vi "HW Run_20201229.vi"(8 "error in (no error)":errorcluster, 11 "ClusterOut in":T1) -> (0 "error out":errorcluster, 3 "ClusterOut out":T1)   [LabVIEW 2018]
uses:
  Controls/HWCluster.ctl
  Controls/Clusts/FPGA_Config_Clust.ctl
  Controls/Enums/TargetNumber.ctl
  Controls/Clusts/AcqData.ctl
  Controls/Clusts/SaturationMonitor.ctl
  Controls/Clusts/FromFPGA_Clust.ctl
  Queue/DataQueueElements.ctl
  Controls/Clusts/TimeDomainData.ctl
  Controls/Enums/LogLoopEnum.ctl
panel:
  out "Target1 2":i32
  out "Elements Remaining 3":u32
  out "Elements Remaining":u32
  out "Target 3":i32
  out "Target1":i32
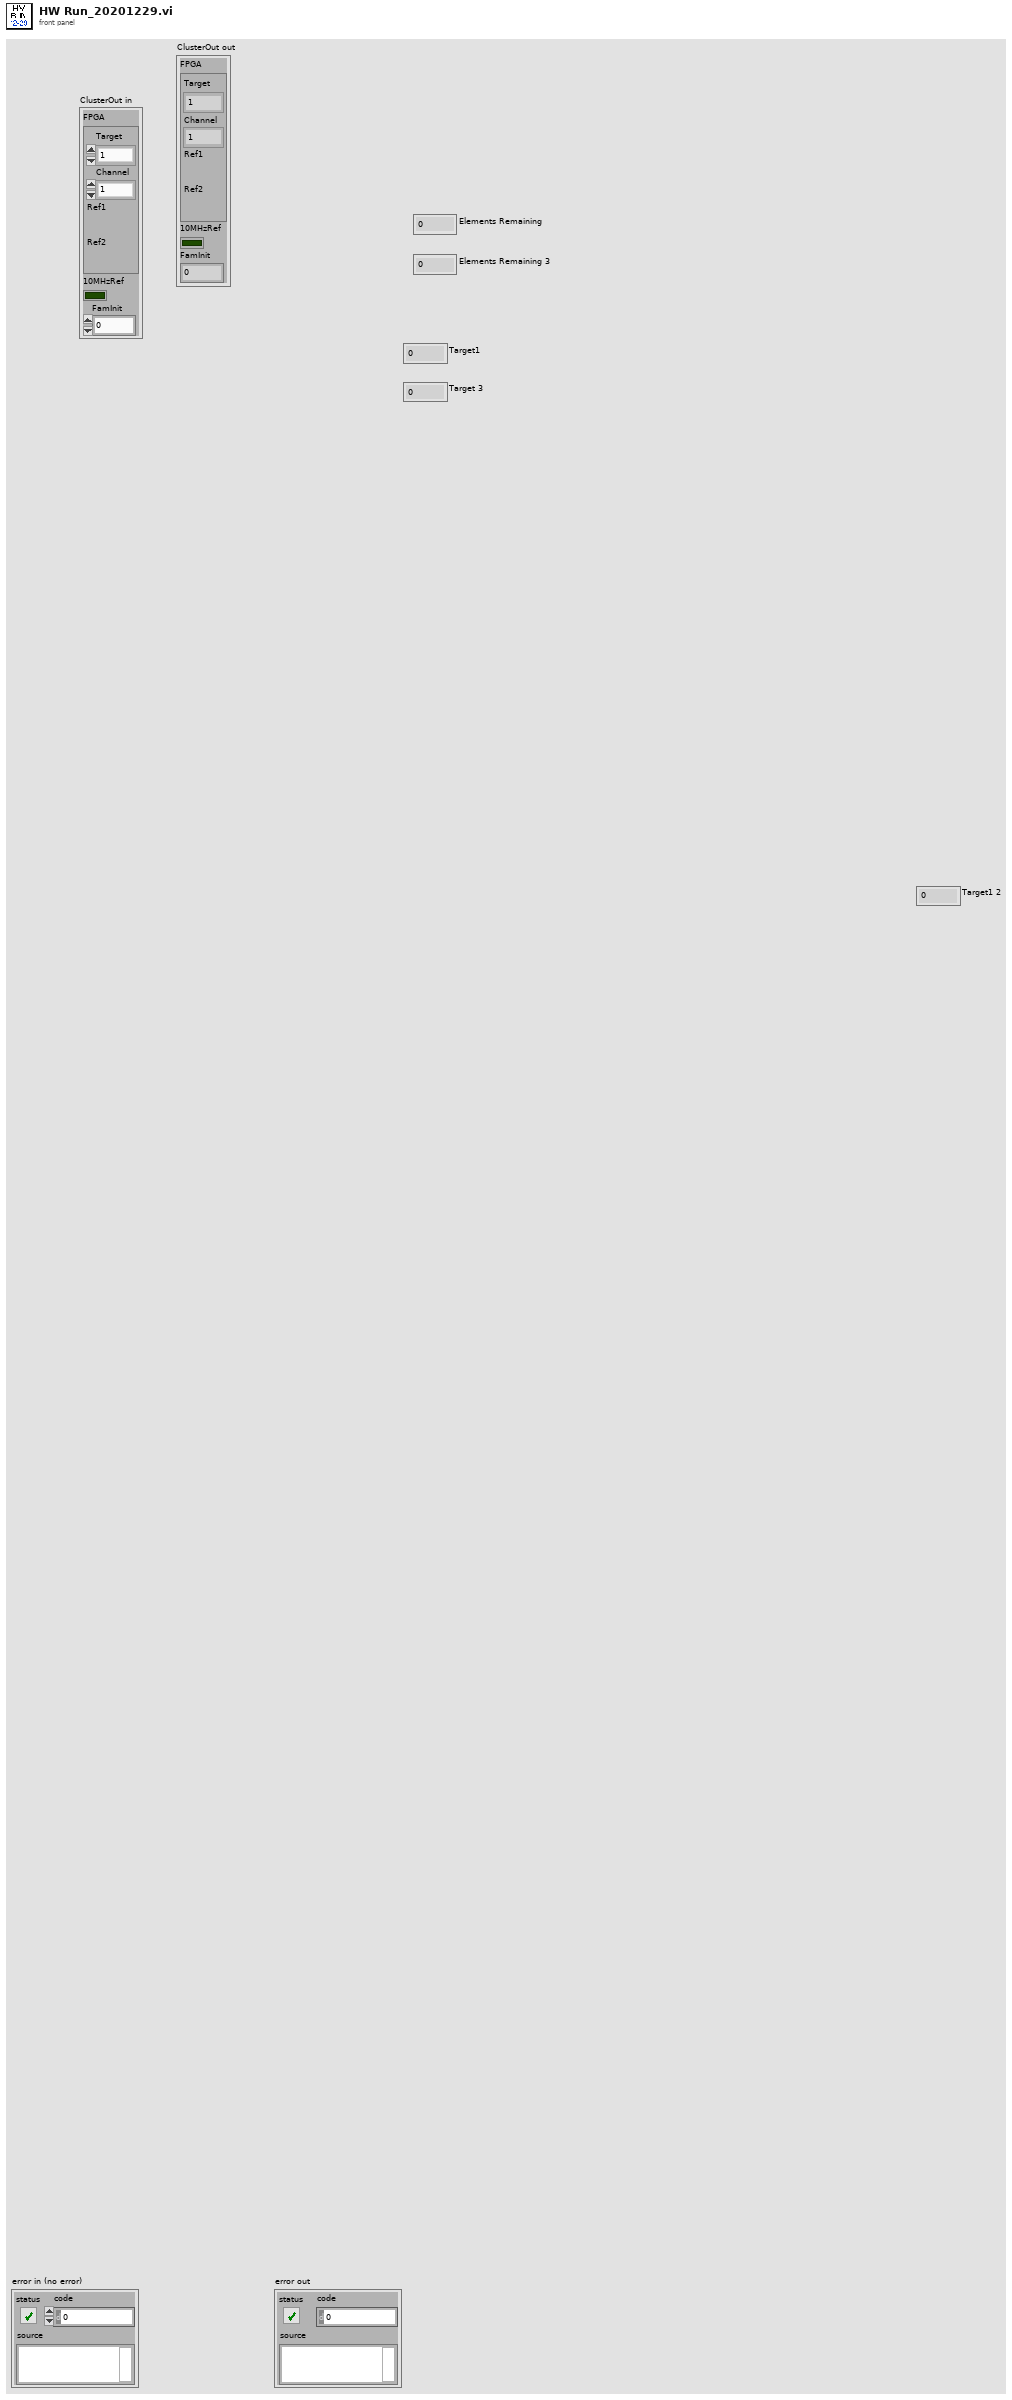
[diagram p1: front panel]
types:
  T1 = typedef "HWCluster.ctl" = cluster{"FPGA":T2, "10MHzRef":bool, "FamInit":i32}
  T2 = typedef "FPGA_Config_Clust.ctl" = cluster{"Target":T3, "Channel":T3, "Ref1":refnum<k20>, "Ref2":refnum<k20>}
  T3 = typedef "TargetNumber.ctl" = enum16{"1", "2", "3", "4"}
  T4 = typedef "AcqData.ctl" = cluster{"Data":fxp<+/-,24,1>[], "#":T3, "Saturat":T5, "FromFPGA":T6, "10MHz":bool}
  T5 = typedef "SaturationMonitor.ctl" = cluster{"MeasMean0":dbl, "MeasMean1":dbl, "MeasMax":dbl, "1_Max":dbl, "4_Max":dbl, "5_Max":dbl, "6_Max":dbl, "7_Max":dbl}
  T6 = typedef "FromFPGA_Clust.ctl" = cluster{"CalTimeDomainI":ext[], "CalTimeDomainI.Index":ext[], "CalTimeDomainQ":ext[], "CalTimeDomainQ.Index":ext[], "BeacTimeDomainI":ext[], "BeacTimeDomainI.Index":ext[], "BeacTimeDomainQ":ext[], "BeacTimeDomainQ.Index":ext[]}
  T7 = typedef "LogLoopEnum.ctl" = enum16{"Log_Init", "Log_Config", "Log_CfgAlarm", "Log_TimeDomain", "Log_Tone", "Log_NoiseTrace", "Log_NoiseSum", "Log_DO", "Log_AI", "Log_TC", "Log_Disdrom", "Log_Weather", "Log_TE", "Log_ADAM", "Log_UPS", "Log_ChkTime", "Log_Alarm", "Log_SSH", "Log_Write", "Log_Exit"}
  T8 = typedef "TimeDomainData.ctl" = cluster{"CalTimeVal":dbl[], "CalTimeCount":u32[], "Enum":T3}
  T9 = typedef "DataQueueElements.ctl" = enum16{"Data_Init", "Data_Config", "Data_AddData", "Data_FreqShift", "Data_FPGA_Write", "Data_Transform", "Data_Send", "Data_Exit"}
  T10 = typedef "Semaphore RefNum" = refnum<k1>
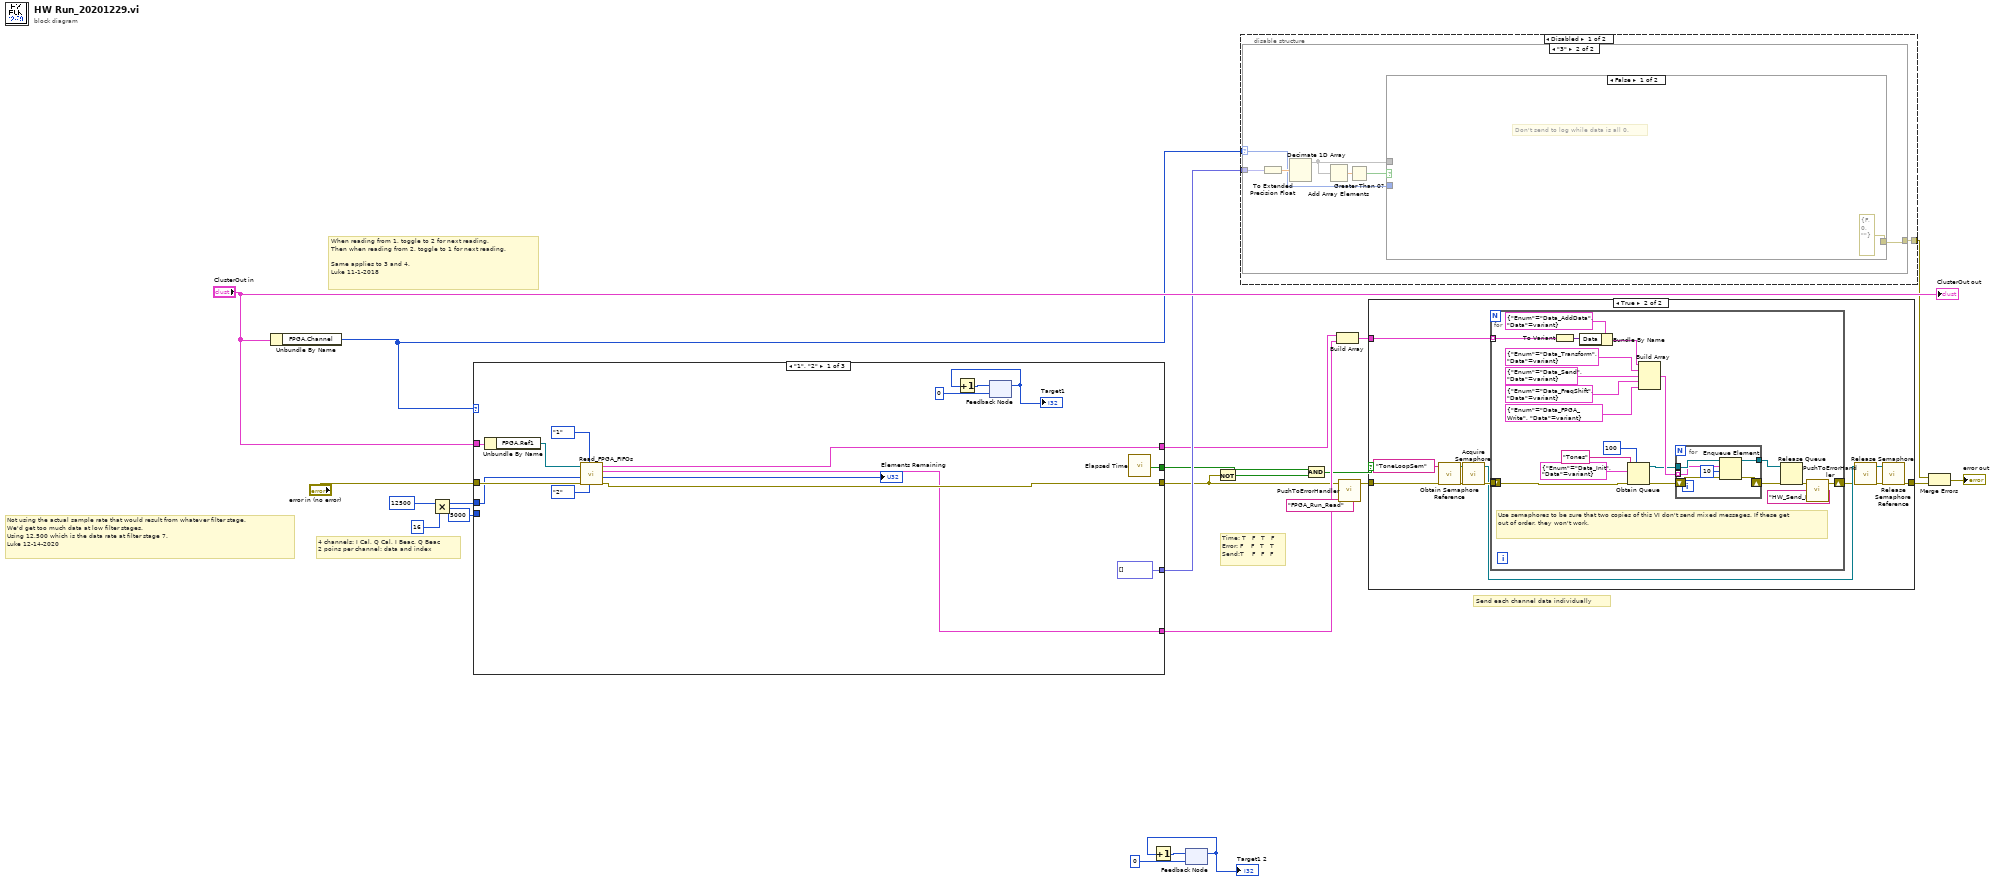
[diagram p0: block diagram]
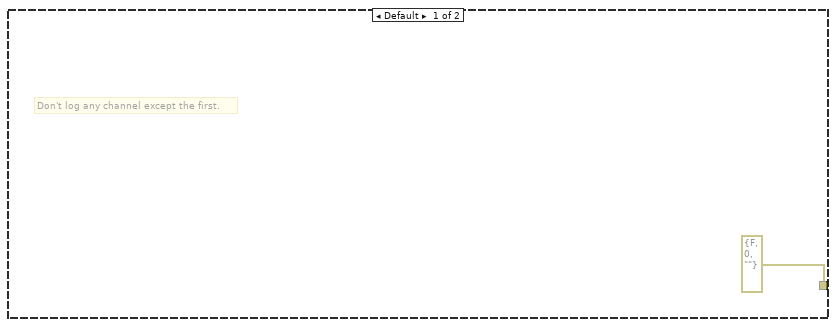
[diagram p3: hidden frame]
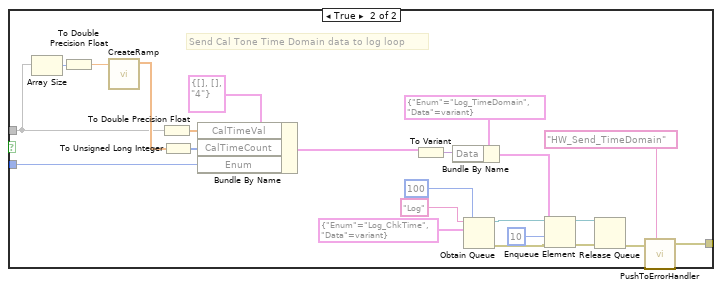
[diagram p4: hidden frame]
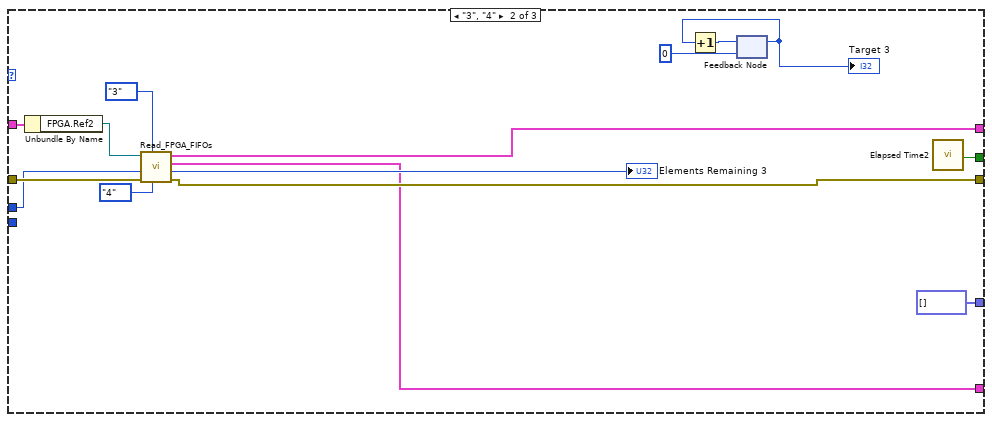
[diagram p6: hidden frame]
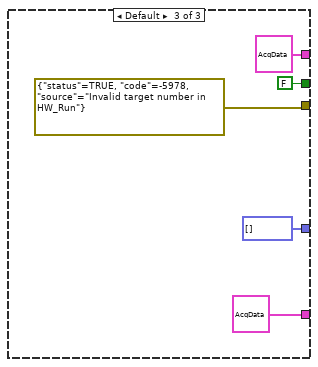
[diagram p7: hidden frame]
diagram:
  # "Time: T   F   T   F\nError: F    F   T   T\nSend:T    F   F   F"
  # "Send each channel data individually"
  # "Not using the actual sample rate that would result from whatever filter stage.\nWe'd get too much data at low filter stages.\nUsing 12,500 which is the data rate at filter stage 7.\nLuke 12-14-2020"
  # "4 channels: I Cal, Q Cal, I Beac, Q Beac\n2 poins per channel: data and index"
  # "When reading from 1, toggle to 2 for next reading.\nThen when reading from 2, toggle to 1 for next reading.\n\nSame applies to 3 and 4. \nLuke 11-1-2018"
  n1 = Unbundle By Name("ClusterOut in") -> ("FPGA.Channel"=w16:T3)
  n2 = Multiply(x=u32 12500, y=u32 16) -> (x*y=w19:u32)
  n3 = case shown="\"1\", \"2\"" w16 {
    tunnel: w19 -> [w30 w46 _]
    tunnel: 5000 ("Timeout (ms)") -> [_ _ _]
    tunnel: "error in (no error)" -> [w32 w48 _]
    tunnel: [fxp<+/-,24,1>[] [] ("Data") fxp<+/-,24,1>[] [] ("Data") fxp<+/-,24,1>[] [] ("Data")] -> w17
    tunnel: [w28 w43 errorcluster {"status"=TRUE, "code"=-5978, "source"="Invalid target number in HW_Run"} ("error out")] -> w1
    tunnel: "ClusterOut in" -> [w38 w53 _]
    tunnel: [w37 w52 FALSE ("Time has Elapsed")] -> w4
    tunnel: [w36 w51 T4 {"Data"=[], "#"=enum."4", "Saturat"={"MeasMean0"=0.0, "MeasMean1"=0.0, "MeasMax"=0.0, "1_Max"=0.0, "4_Max"=0.0, "5_Max"=0.0, "6_Max"=0.0, "7_Max"=0.0}, "FromFPGA"={"CalTimeDomainI"=[], "CalTimeDomainI.Index"=[], "CalTimeDomainQ"=[], "CalTimeDomainQ.Index"=[], "BeacTimeDomainI"=[], "BeacTimeDomainI.Index"=[], "BeacTimeDomainQ"=[], "BeacTimeDomainQ.Index"=[]}, "10MHz"=FALSE} ("AcqData")] -> w13
    tunnel: [w24 w40 T4 {"Data"=[], "#"=enum."4", "Saturat"={"MeasMean0"=0.0, "MeasMean1"=0.0, "MeasMax"=0.0, "1_Max"=0.0, "4_Max"=0.0, "5_Max"=0.0, "6_Max"=0.0, "7_Max"=0.0}, "FromFPGA"={"CalTimeDomainI"=[], "CalTimeDomainI.Index"=[], "CalTimeDomainQ"=[], "CalTimeDomainQ.Index"=[], "BeacTimeDomainI"=[], "BeacTimeDomainI.Index"=[], "BeacTimeDomainQ"=[], "BeacTimeDomainQ.Index"=[]}, "10MHz"=FALSE}] -> w10
    frame "1", "2" {
      n4 = Unbundle By Name(w38) -> ("FPGA.Ref1"=w31:refnum<k20>)
      n5 = call "Read_FPGA_FIFOs.vi"("TargetB"=TargetNumber."2", "TargetA"=TargetNumber."1" ("Target"), "error in"=w32, "#Elements"=w30, "FPGA VI Ref"=w31) -> ("error out"=w28:errorcluster, "Elements Remaining"=→"Elements Remaining":u32, "AcqDataB"=w24:T4, "AcqDataA"=w36:T4)  [unwired: 3 in]
      n6 = feedback #1(0) -> (w27:i32)
      "Target1" <- w27
      n7 = Increment(x=w27) -> (x+1=w35:i32)
      n8 = feedback-in #1(w35) -> ()
      n9 = call "Elapsed Time"() -> ("Time has Elapsed"=w37:bool)  [unwired: 12 in, 7 out]
    }
    frame "3", "4" {
      n10 = Unbundle By Name(w53) -> ("FPGA.Ref2"=w47:refnum<k20>)
      n11 = call "Read_FPGA_FIFOs.vi"("TargetB"=TargetNumber."4", "TargetA"=TargetNumber."3" ("Target"), "error in"=w48, "#Elements"=w46, "FPGA VI Ref"=w47) -> ("error out"=w43:errorcluster, "Elements Remaining"=→"Elements Remaining 3":u32, "AcqDataB"=w40:T4, "AcqDataA"=w51:T4)  [unwired: 3 in]
      n12 = feedback #2(0) -> (w42:i32)
      "Target 3" <- w42
      n13 = Increment(x=w42) -> (x+1=w50:i32)
      n14 = feedback-in #2(w50) -> ()
      n15 = call "Elapsed Time2"() -> ("Time has Elapsed"=w52:bool)  [unwired: 12 in, 7 out]
    }
    frame Default {
    }
  }
  n16 = feedback #3(0) -> (w9:i32)
  "Target1 2" <- w9
  n17 = Increment(x=w9) -> (x+1=w7:i32)
  n18 = feedback-in #3(w7) -> ()
  n19 = Not(x=w1) -> (.not. x?=w2:bool)
  n20 = disable-structure shown="Disabled" {
    disable-tunnel: w17 -> [w61 _]
    disable-tunnel: w16 -> [w60 _]
    disable-tunnel: [w59 _] -> w14
    frame Disabled {
      n21 = case shown="\"3\"" w60 {
        selector: w60 -> [_ w68]
        tunnel: w61 -> [_ w67]
        tunnel: [errorcluster {"status"=FALSE, "code"=0, "source"=""} ("ErrorOut") w66] -> w59
        frame Default {
          # "Don't log any channel except the first."
        }
        frame "3" {
          n22 = To Extended Precision Float(1:w67) -> (0:w69:ext[])
          n23 = Decimate 1D Array(w69) -> (w63:ext[])  [unwired: 3 out]
          n24 = Add Array Elements(numeric array=w63) -> (sum=w65:ext)
          n25 = Greater Than 0?(x=w65) -> (x > 0?=w64:bool)
          n26 = case shown="False" w64 {
            tunnel: w68 -> [_ w91]
            tunnel: [errorcluster {"status"=FALSE, "code"=0, "source"=""} ("ErrorOut") w74] -> w66
            tunnel: w63 -> [_ w72]
            frame False {
              # "Don't send to log while data is all 0."
            }
            frame True {
              # "Send Cal Tone Time Domain data to log loop"
              n27 = Array Size(array=w72) -> (size(s)=w89:i32)
              n28 = To Double Precision Float(number=w89) -> (double precision float=w87:dbl)
              n29 = call "CreateRamp.vi"("ArraySize"=w87) -> ("Ramp Pattern"=w88:dbl[])  [unwired: 10 in]
              n30 = To Double Precision Float(number=w72) -> (double precision float=w92:dbl[])
              n31 = To Unsigned Long Integer(number=w88) -> (unsigned 32bit integer=w90:u32[])
              n32 = Bundle By Name(cluster=T8 {"CalTimeVal"=[], "CalTimeCount"=[], "Enum"=enum."4"} ("TimeDomain"), "CalTimeVal"=w92, "CalTimeCount"=w90, "Enum"=w91) -> (w79:T8)
              n33 = To Variant(anything=w79) -> (Variant=w80:variant)
              n34 = Bundle By Name(cluster=cluster{"Enum":T7, "Data":variant} {"Enum"=enum."Log_TimeDomain", "Data"=variant} ("element"), "Data"=w80) -> (w81:cluster{"Enum":T7, "Data":variant})
              n35 = Obtain Queue(max queue size (-1, unlimited)=100, name (unnamed)="Log", element data type=cluster{"Enum":T7, "Data":variant} {"Enum"=enum."Log_ChkTime", "Data"=variant}) -> (queue out=w84:refnum<queue>, error out=w78:errorcluster)  [unwired: 2 in, 1 out]
              n36 = Enqueue Element(queue=w84, element=w81, timeout in ms (-1)=10, error in (no error)=w78) -> (queue out=w77:refnum<queue>, error out=w76:errorcluster)  [unwired: 1 out]
              n37 = Release Queue(queue=w77, error in (no error)=w76) -> (error out=w75:errorcluster)  [unwired: 1 in, 2 out]
              n38 = call "PushToErrorHandler.vi"("ErrorIn"=w75, "ErrorLocation"="HW_Send_TimeDomain") -> ("ErrorOut"=w74:errorcluster)  [unwired: 5 in]
            }
          }
        }
      }
    }
    frame Enabled {
    }
  }
  n39 = Compound Arithmetic op=AND(w4, w2) -> (w3:bool)
  n40 = Build Array(w13, w10) -> (w11:T4[])
  n41 = call "PushToErrorHandler.vi"("ErrorIn"=w1, "ErrorLocation"="FPGA_Run_Read") -> ("ErrorOut"=w6:errorcluster)  [unwired: 5 in]
  n42 = case shown="True" w3 {
    tunnel: [w94 w96] -> w22
    tunnel: w6 -> [w94 w100]
    tunnel: w11 -> [_ w105]
    frame False {
    }
    frame True {
      n43 = call <vilib>:"Obtain Semaphore Reference.vi"("error in (no error)"=w100, "name (unnamed)"="ToneLoopSem") -> ("error out"=w104:errorcluster, "semaphore"=w103:T10)  [unwired: 3 in, 1 out]
      n44 = call <vilib>:"Acquire Semaphore.vi"("error in (no error)"=w104, "semaphore"=w103) -> ("error out"=w101:errorcluster, "semaphore out"=w99:T10)  [unwired: 3 in, 1 out]
      n45 = for {
        tunnel: w105 -> [w110] mode=indexing
        shift-right: [w106] -> w98
        shift-left: _ -> [_]
        tunnel: w101 -> [w109]
        # "Use semaphores to be sure that two copies of this VI don't send mixed messages. If these get out of order, they won't work."
        n46 = To Variant(anything=w110) -> (Variant=w120:variant)
        n47 = Bundle By Name(cluster=cluster{"Enum":T9, "Data":variant} {"Enum"=enum."Data_AddData", "Data"=variant}, "Data"=w120) -> (w119:cluster{"Enum":T9, "Data":variant})
        n48 = Obtain Queue(max queue size (-1, unlimited)=100, name (unnamed)="Tones", element data type=cluster{"Enum":T9, "Data":variant} {"Enum"=enum."Data_Init", "Data"=variant}, error in (no error)=w109) -> (queue out=w114:refnum<queue>, error out=w113:errorcluster)  [unwired: 1 in, 1 out]
        n49 = Build Array(w119, cluster{"Enum":T9, "Data":variant} {"Enum"=enum."Data_Transform", "Data"=variant}, cluster{"Enum":T9, "Data":variant} {"Enum"=enum."Data_Send", "Data"=variant}, cluster{"Enum":T9, "Data":variant} {"Enum"=enum."Data_FreqShift", "Data"=variant}, cluster{"Enum":T9, "Data":variant} {"Enum"=enum."Data_FPGA_Write", "Data"=variant}) -> (w125:cluster{"Enum":T9, "Data":variant}[])
        n50 = for {
          tunnel: w114 -> [w129]
          tunnel: w125 -> [w128] mode=indexing
          shift-right: [w130] -> w108
          shift-left: w113 -> [w131]
          tunnel: [w127] -> w112
          n51 = Enqueue Element(queue=w129, element=w128, timeout in ms (-1)=10, error in (no error)=w131) -> (queue out=w127:refnum<queue>, error out=w130:errorcluster)  [unwired: 1 out]
        }
        n52 = Release Queue(queue=w112, error in (no error)=w108) -> (error out=w107:errorcluster)  [unwired: 1 in, 2 out]
        n53 = call "PushToErrorHandler.vi"("ErrorIn"=w107, "ErrorLocation"="HW_Send_Data") -> ("ErrorOut"=w106:errorcluster)  [unwired: 5 in]
      }
      n54 = call <vilib>:"Release Semaphore.vi"("error in (no error)"=w98, "semaphore"=w99) -> ("error out"=w97:errorcluster, "semaphore out"=w95:T10)  [unwired: 4 in]
      n55 = call <vilib>:"Release Semaphore Reference.vi"("error in (no error)"=w97, "semaphore"=w95) -> ("error out"=w96:errorcluster)  [unwired: 8 in, 1 out]
    }
  }
  n56 = Merge Errors(w14, w22) -> (→"error out":errorcluster)
  "ClusterOut out" <- "ClusterOut in"
